vi "nth Derivative of Rational Polynomial (CDB).vi"(9 "order":i32, 10 "Q(x)":cdb[](array[numeric]) format="%#.2g", 11 "P(x)":cdb[](array[numeric]) format="%#.2g") -> (0 "error":i32, 2 "Denominator d[P(x)/Q(x)]/dx":cdb[](array[numeric]) format="%#.2g", 3 "Numerator d[P(x)/Q(x)]/dx":cdb[](array[numeric]) format="%#.2g")   [LabVIEW 2010, in "NI_AALPro.lvlib"]
doc: "Calculates the nth order derivative of a rational polynomial. The data types you wire to the <B>P(x)</B> and <B>Q(x)</B> inputs determine the polymorphic instance to use."
uses:
  NI_AALPro.lvlib
  Remove Zero Coefficients (CDB).vi
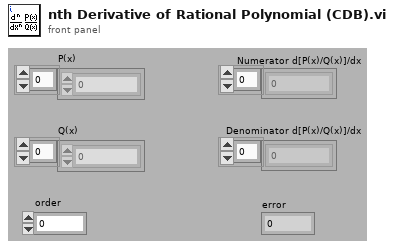
[diagram p1: front panel]
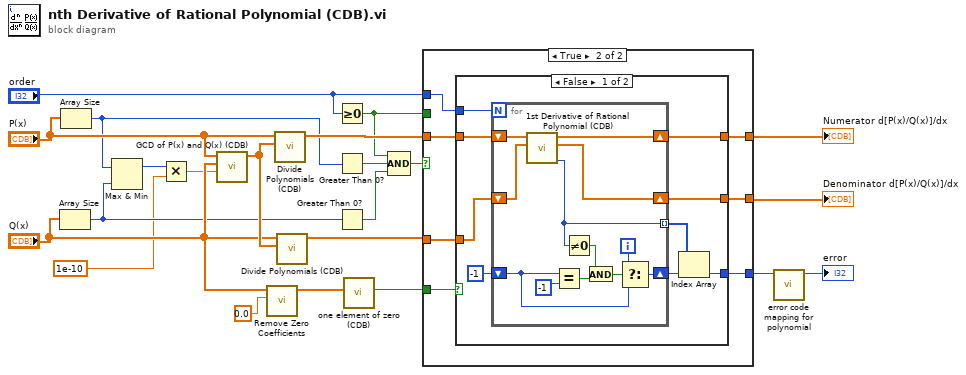
[diagram p0: block diagram]
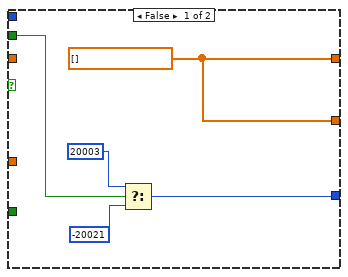
[diagram p2: hidden frame]
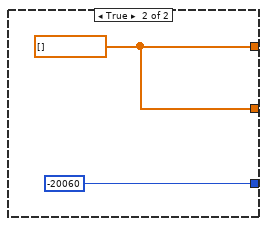
[diagram p3: hidden frame]
diagram:
  n1 = Array Size(array="Q(x)") -> (size(s)=w9:i32)
  n2 = Array Size(array="P(x)") -> (size(s)=w10:i32)
  n3 = Max & Min(x=w10, y=w9) -> (max(x,y)=w8:i32)  [unwired: 1 out]
  n4 = Multiply(x=w8, y=1e-10 ("eps for nth div of p/q")) -> (x*y=w3:dbl)
  n5 = call "GCD of P(x) and Q(x) (CDB).vi"("tolerance"=w3, "Q(x)"="Q(x)", "P(x)"="P(x)") -> ("Greatest Common Divisor"=w22:cdb[])  [unwired: 7 in, 1 out]
  n6 = call-poly "Remove Zero Coefficients.vi"("threshold"=0.0, "P(x) In"="Q(x)") -> ("P(x) Out"=w6:cdb[])  [unwired: 7 in, 2 out]
  n7 = call "Divide Polynomials (CDB).vi"("Q(x)"=w22, "P(x)"="P(x)") -> ("P(x)/Q(x)"=w21:cdb[])  [unwired: 7 in, 2 out]
  n8 = call "Divide Polynomials (CDB).vi"("Q(x)"=w22, "P(x)"="Q(x)") -> ("P(x)/Q(x)"=w20:cdb[])  [unwired: 7 in, 2 out]
  n9 = Greater Or Equal To 0?(x="order") -> (x >= 0?=w4:bool)
  n10 = Greater Than 0?(x=w10) -> (x > 0?=w15:bool)
  n11 = Greater Than 0?(x=w9) -> (x > 0?=w14:bool)
  n12 = call "one element of zero (CDB).vi"("Array in"=w6) -> ("equal [0]?"=w5:bool)  [unwired: 10 in]
  n13 = Compound Arithmetic op=AND(w4, w15, w14) -> (w13:bool)
  n14 = case shown="True" w13 {
    tunnel: w21 -> [_ w34]
    tunnel: "order" -> [_ w30]
    tunnel: [w27 w33] -> w19
    tunnel: w20 -> [_ w32]
    tunnel: [w27 w31] -> w18
    tunnel: w5 -> [_ w29]
    tunnel: w4 -> [w26 _]
    tunnel: [w23 w28] -> w2
    frame False {
      w27 = cdb[] [] ("Numerator d[p(s)/q(s)]/ds")
      n15 = Select(t=20003 ("empty array"), s=w26, f=-20021 ("minus order")) -> (s? t:f=w23:i32)
    }
    frame True {
      n16 = case shown="False" w29 {
        tunnel: w34 -> [w43 _]
        tunnel: [w42 w57] -> w33
        tunnel: w32 -> [w41 _]
        tunnel: [w40 w57] -> w31
        tunnel: w30 -> [w39 _]
        tunnel: [w35 -20060 ("divide by zero")] -> w28
        frame False {
          n17 = for {
            N: w39 -> [_]
            shift-right: [w53] -> w42
            shift-left: w43 -> [w55]
            shift-right: [w52] -> w40
            shift-left: w41 -> [w54]
            shift-right: [w45] -> w37
            shift-left: -1 -> [w46]
            tunnel: [w44] -> w36 mode=indexing
            i -> [w47]
            n18 = call "1st Derivative of Rational Polynomial (CDB).vi"("Q(x)"=w54, "P(x)"=w55) -> ("error"=w44:i32, "Denominator d[P(x)/Q(x)]/dx"=w52:cdb[], "Numerator d[P(x)/Q(x)]/dx"=w53:cdb[])  [unwired: 7 in]
            n19 = Equal?(x=w46, y=-1) -> (x = y?=w50:bool)
            n20 = Not Equal To 0?(x=w44) -> (x != 0?=w49:bool)
            n21 = And(x=w49, y=w50) -> (x .and. y?=w48:bool)
            n22 = Select(t=w47, s=w48, f=w46) -> (s? t:f=w45:i32)
          }
          n23 = Index Array(array=w36, index=w37) -> (element=w35:i32)
        }
        frame True {
          w57 = cdb[] [] ("CDB")
        }
      }
    }
  }
  "Denominator d[P(x)/Q(x)]/dx" <- w18
  "Numerator d[P(x)/Q(x)]/dx" <- w19
  n24 = call "error code mapping for polynomial.vi"("error in"=w2) -> ("error out"=→"error":i32)  [unwired: 10 in]
